vi "DHE_ReadTimingFromFile.vi"(8 "error in (no error)":errorcluster, 11 "configfile":path) -> (0 "error out":errorcluster, 2 "timeout offset":i32=30000)   [LabVIEW 2016]
uses:
  <vilib>/Utility/config.llb/Read Key (String).vi
  <vilib>/Utility/config.llb/NI_LVConfig.lvlib
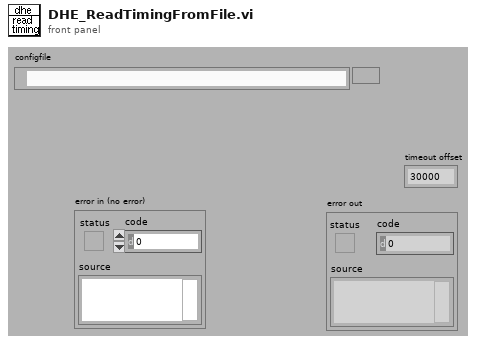
[diagram p1: front panel]
types:
  T1 = typedef "DatabaseHand_RefNum.ctl" = refnum<vi>
  T2 = typedef "NI_LVConfig.lvlib/Config Data RefNum.ctl" = refnum<k1>
  T3 = typedef "CMN_TimingInfo.ctl" = cluster{"PixelTime":sgl, "SkipPixel":sgl, "SkipRow":sgl, "ShiftRow":sgl, "ShiftedPix":u16, "known_overhead":sgl, "DET_READ_TIME":sgl}
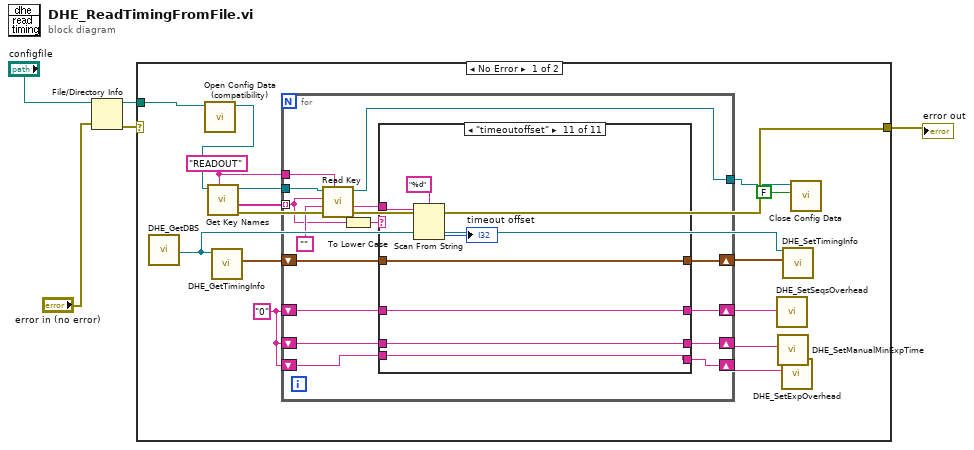
[diagram p0: block diagram]
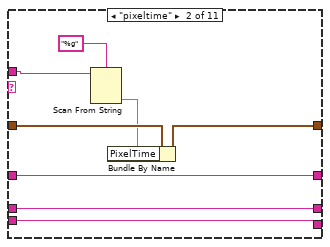
[diagram p3: hidden frame]
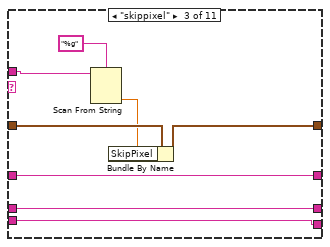
[diagram p4: hidden frame]
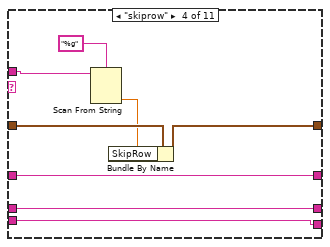
[diagram p5: hidden frame]
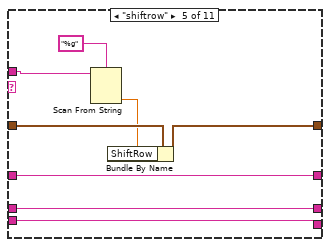
[diagram p6: hidden frame]
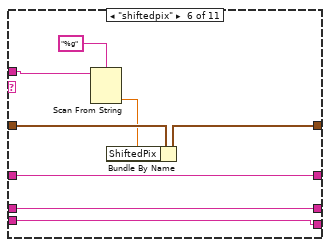
[diagram p7: hidden frame]
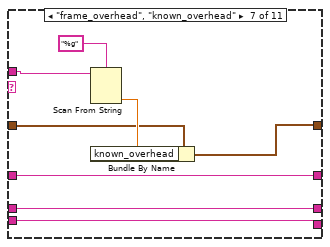
[diagram p8: hidden frame]
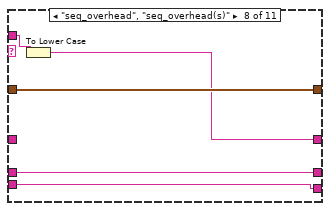
[diagram p9: hidden frame]
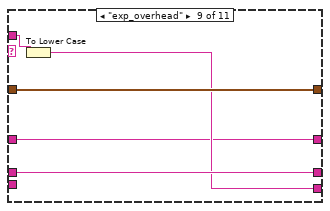
[diagram p10: hidden frame]
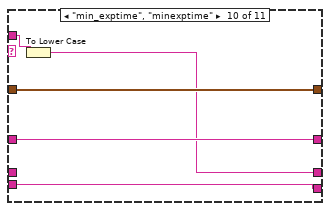
[diagram p11: hidden frame]
diagram:
  n1 = File/Directory Info(path="configfile", error in="error in (no error)") -> (path out=w1:path, error out=w4:errorcluster)  [unwired: 5 out]
  n2 = case shown="No Error" w4 {
    selector: w4 -> [_ w110]
    tunnel: [w14 w110] -> w3
    tunnel: w1 -> [w20 _]
    frame No Error {
      w9 = "0"
      w16 = "READOUT" ("section")
      n3 = call "DHE_GetDBS.vi"() -> ("DHE_DBSRef"=w12:T1)  [unwired: 9 out]
      n4 = call <vilib>:"Open Config Data (compatibility).vi"("configuration file path"=w20) -> ("refnum"=w19:T2)  [unwired: 8 in, 2 out]
      n5 = call <vilib>:"Get Key Names.vi"("section"=w16, "refnum"=w19) -> ("error out"=w14:errorcluster, "key names"=w18:string[], "refnum out"=w17:T2)  [unwired: 1 in, 6 out]
      n6 = call "DHE_GetTimingInfo.vi"("Database RefNum out"=w12) -> ("Timing"=w15:T3)  [unwired: 10 out]
      n7 = for {
        tunnel: w18 -> [w28] mode=indexing
        tunnel: w17 -> [w35]
        tunnel: w16 -> [w34]
        shift-right: [w30] -> w13
        shift-left: w15 -> [w31]
        shift-right: [w26] -> w11
        shift-left: w9 -> [w27]
        shift-right: [w24] -> w10
        shift-left: w9 -> [w25]
        shift-right: [w23] -> w8
        shift-left: w9 -> [w22]
        tunnel: [w21] -> w7
        n8 = call-poly <vilib>:"Read Key.vi"("section"=w34, "default value"="", "key"=w28, "refnum"=w35) -> ("value"=w32:string, "refnum out"=w21:T2)  [unwired: 2 in, 4 out]
        n9 = To Lower Case(string=w28) -> (all lower case string=w33:string)
        n10 = case shown="\"timeoutoffset\"" w33 {
          tunnel: w32 -> [_ w45 w53 w61 w69 w77 w87 w91 w96 w101 w105]
          tunnel: w31 -> [w39 w47 w55 w63 w71 w79 w84 w92 w97 w102 w109]
          tunnel: [w39 w46 w54 w62 w70 w78 w83 w92 w97 w102 w109] -> w30
          tunnel: w27 -> [w38 w42 w50 w58 w66 w74 w82 _ w93 w100 w108]
          tunnel: [w38 w42 w50 w58 w66 w74 w82 w90 w93 w100 w108] -> w26
          tunnel: w25 -> [w37 w41 w49 w57 w65 w73 w81 w89 w95 _ w106]
          tunnel: [w37 w41 w49 w57 w65 w73 w81 w89 w95 w99 w106] -> w24
          tunnel: [w36 w40 w48 w56 w64 w72 w80 w88 w94 w98 w107] -> w23
          tunnel: w22 -> [w36 w40 w48 w56 w64 w72 w80 w88 _ w98 w107]
          frame Default {
          }
          frame "pixeltime" {
            n11 = Scan From String(format string="%g", input string=w45) -> (output 1=w43:dbl)  [unwired: 2 in, 4 out]
            n12 = Bundle By Name(cluster=w47, "PixelTime"=w43) -> (w46:T3)
          }
          frame "skippixel" {
            n13 = Scan From String(format string="%g", input string=w53) -> (output 1=w51:dbl)  [unwired: 2 in, 4 out]
            n14 = Bundle By Name(cluster=w55, "SkipPixel"=w51) -> (w54:T3)
          }
          frame "skiprow" {
            n15 = Scan From String(format string="%g", input string=w61) -> (output 1=w59:dbl)  [unwired: 2 in, 4 out]
            n16 = Bundle By Name(cluster=w63, "SkipRow"=w59) -> (w62:T3)
          }
          frame "shiftrow" {
            n17 = Scan From String(format string="%g", input string=w69) -> (output 1=w67:dbl)  [unwired: 2 in, 4 out]
            n18 = Bundle By Name(cluster=w71, "ShiftRow"=w67) -> (w70:T3)
          }
          frame "shiftedpix" {
            n19 = Scan From String(format string="%g", input string=w77) -> (output 1=w75:dbl)  [unwired: 2 in, 4 out]
            n20 = Bundle By Name(cluster=w79, "ShiftedPix"=w75) -> (w78:T3)
          }
          frame "frame_overhead", "known_overhead" {
            n21 = Scan From String(format string="%g", input string=w87) -> (output 1=w85:dbl)  [unwired: 2 in, 4 out]
            n22 = Bundle By Name(cluster=w84, "known_overhead"=w85) -> (w83:T3)
          }
          frame "seq_overhead", "seq_overhead(s)" {
            n23 = To Lower Case(string=w91) -> (all lower case string=w90:string)
          }
          frame "exp_overhead" {
            n24 = To Lower Case(string=w96) -> (all lower case string=w94:string)
          }
          frame "min_exptime", "minexptime" {
            n25 = To Lower Case(string=w101) -> (all lower case string=w99:string)
          }
          frame "timeoutoffset" {
            n26 = Scan From String(format string="%d", input string=w105) -> (output 1=→"timeout offset":i32)  [unwired: 2 in, 4 out]
          }
        }
      }
      n27 = call "DHE_SetSeqsOverhead.vi"("SeqsOverhead"=w11) -> ()  [unwired: 11 out]
      n28 = call "DHE_SetManualMinExpTime.vi"("ManualMinExptime"=w10) -> ()  [unwired: 11 out]
      n29 = call "DHE_SetExpOverhead.vi"("ExpOverhead"=w8) -> ()  [unwired: 11 out]
      n30 = call "DHE_SetTimingInfo.vi"("Timing"=w13, "Database RefNum out"=w12) -> ()  [unwired: 10 out]
      n31 = call <vilib>:"Close Config Data.vi"("write file if changed (T)"=FALSE ("write configuration file? (T)"), "refnum"=w7) -> ()  [unwired: 1 in, 9 out]
    }
    frame Error {
    }
  }
  "error out" <- w3
